vi "Control - Closed Loop Throttle.vi"(7 "Fresh Air Mass [mg/cyc]":sgl, 8 "Control Inputs":T1={"Engine Speed [RPM]"=0.0, "Engine Status"=enum."STALLED", "Load Control \nMode"=enum."High-Idle Governor", "dt(s)"=0.0, "Number of Cylinders"=0, "Engine Displacement [cc]"=0.0, "StoichAFR"=0.0, "Q.LHV Fuel [kJ/kg]"=0.0, "BattV PSU [V]"=0.0, "12V PSU [V]"=0.0, "5V PSU [V]"=0.0, "Pedal Position [%]"=0.0, "Oil Pressure [kPa]"=0.0, "Oil Temp [C]"=0.0, "Oil Level [%]"=0.0, "Engine Coolant Temp (ECT) [C]"=0.0, "Engine Coolant Pressure [kPa]"=0.0, "Rail Pressure [bar]"=0.0, "Fuel Pressure [kPa]"=0.0, "Fuel Temp [C]"=0.0, "Vacuum Pressure [kPa]"=0.0, "Throttle Position [%]"=0.0, "Cam1 Advance [CAD]"=0.0, "Cam2 Advance [CAD]"=0.0, "Cam3 Advance [CAD]"=0.0, "Cam4 Advance [CAD]"=0.0, "CA50 Control Output [CAD]"=[], "CA50 Control Output Valid"=[], "Intake Air Temp (IAT) [C]"=0.0, "Barometric Air Pressure [kPa]"=0.0, "Intake Air Rel. Humidity [%]"=0.0, "Mass Air Flow (MAF) [kg/hr]"=0.0, "Turbo Inlet Air Pressure [kPa]"=0.0, "Turbo Inlet Air Temp [C]"=0.0, "Turbo Outlet Air Pressure [kPa]"=0.0, "Turbo Outlet Air Temp [C]"=0.0, "CAC Outlet Pressure [kPa]"=0.0, "CAC Outlet Temp [C]"=0.0, "Intake Manifold Pressure (MAP) [kPa]"=0.0, "Intake Manifold Temp (MAT) [C]"=0.0, "Exhaust Manifold Pressure [kPa]"=0.0, "Exhaust Manifold Temp [C]"=0.0, "HighP EGR Cooler Outlet Pressure [kPa]"=0.0, "HighP EGR Cooler Outlet Temp [C]"=0.0, "HighP EGR Differential Pressure [kPa]"=0.0, "HighP EGR Valve Position [%]"=0.0, "Turbo Outlet Exhaust Pressure [kPa]"=0.0, "Turbo Outlet Exhaust Temp [C]"=0.0, "VGT Position 1 [%]"=0.0, "VGT Position 2 [%]"=0.0, "Turbo Speed 1 [RPM]"=0.0, "Turbo Speed 2 [RPM]"=0.0, "LowP EGR Differential Pressure [kPa]"=0.0, "LowP EGR Valve Position [%]"=0.0, "UEGO1Lambda"=0.0, "UEGO1_Hot"=FALSE, "UEGO2Lambda"=0.0, "UEGO2_Hot"=FALSE, "Knock Intensity"=[], "Knock"=[]} {"Knock Intensity" format="%.2f"; "CA50 Control Output [CAD]" format="%.2f"; "Exhaust Manifold Temp [C]" format="%#_6f"; "UEGO2Lambda" format="%.2f"; "Intake Manifold Temp (MAT) [C]" format="%#_6f"; "UEGO1Lambda" format="%.2f"}, 9 "Pedal [%]":sgl, 10 "Intake MAP Desired [kPa]":sgl, 11 "Fresh Air Mass Desired [mg/cyc]":sgl) -> (3 "Throttle Position [%Open]":sgl)   [LabVIEW 2015, in "ECS-RT.lvlib"]
uses:
  ECS-RT.lvlib
  Typedefs/Control Inputs/Control Inputs.ctl
  Typedefs/EPT/Engine Status.ctl
  Typedefs/MISC/Load Control Mode.ctl
  ECS-Shared.lvlib
panel:
  out "Pratio":sgl
  out "B1":sgl
  out "A1":sgl
  out "Pcr":sgl
  out "Psi":sgl
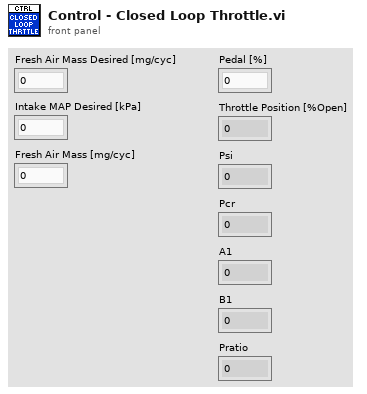
[diagram p1: front panel]
types:
  T1 = typedef "ECS-Shared.lvlib/Control Inputs.ctl" = cluster{"Engine Speed [RPM]":sgl, "Engine Status":T2, "Load Control \nMode":T3, "dt(s)":sgl, "Number of Cylinders":u8, "Engine Displacement [cc]":sgl, "StoichAFR":sgl, "Q.LHV Fuel [kJ/kg]":sgl, "BattV PSU [V]":sgl, "12V PSU [V]":sgl, "5V PSU [V]":sgl, "Pedal Position [%]":sgl, "Oil Pressure [kPa]":sgl, "Oil Temp [C]":sgl, "Oil Level [%]":sgl, "Engine Coolant Temp (ECT) [C]":sgl, "Engine Coolant Pressure [kPa]":sgl, "Rail Pressure [bar]":sgl, "Fuel Pressure [kPa]":sgl, "Fuel Temp [C]":sgl, "Vacuum Pressure [kPa]":sgl, "Throttle Position [%]":sgl, "Cam1 Advance [CAD]":sgl, "Cam2 Advance [CAD]":sgl, "Cam3 Advance [CAD]":sgl, "Cam4 Advance [CAD]":sgl, "CA50 Control Output [CAD]":sgl[], "CA50 Control Output Valid":bool[], "Intake Air Temp (IAT) [C]":sgl, "Barometric Air Pressure [kPa]":sgl, "Intake Air Rel. Humidity [%]":sgl, "Mass Air Flow (MAF) [kg/hr]":sgl, "Turbo Inlet Air Pressure [kPa]":sgl, "Turbo Inlet Air Temp [C]":sgl, "Turbo Outlet Air Pressure [kPa]":sgl, "Turbo Outlet Air Temp [C]":sgl, "CAC Outlet Pressure [kPa]":sgl, "CAC Outlet Temp [C]":sgl, "Intake Manifold Pressure (MAP) [kPa]":sgl, "Intake Manifold Temp (MAT) [C]":sgl, "Exhaust Manifold Pressure [kPa]":sgl, "Exhaust Manifold Temp [C]":sgl, "HighP EGR Cooler Outlet Pressure [kPa]":sgl, "HighP EGR Cooler Outlet Temp [C]":sgl, "HighP EGR Differential Pressure [kPa]":sgl, "HighP EGR Valve Position [%]":sgl, "Turbo Outlet Exhaust Pressure [kPa]":sgl, "Turbo Outlet Exhaust Temp [C]":sgl, "VGT Position 1 [%]":sgl, "VGT Position 2 [%]":sgl, "Turbo Speed 1 [RPM]":sgl, "Turbo Speed 2 [RPM]":sgl, "LowP EGR Differential Pressure [kPa]":sgl, "LowP EGR Valve Position [%]":sgl, "UEGO1Lambda":sgl, "UEGO1_Hot":bool, "UEGO2Lambda":sgl, "UEGO2_Hot":bool, "Knock Intensity":sgl[], "Knock":bool[]}
  T2 = typedef "ECS-Shared.lvlib/Engine Status.ctl" = enum16{"OFF", "STALLED", "CRANKING", "RUNNING", "ACCEL", "DECEL", "SAFE"}
  T3 = typedef "ECS-Shared.lvlib/Load Control Mode.ctl" = enum16{"No Governor", "Low-Idle Governor", "High-Idle Governor"}
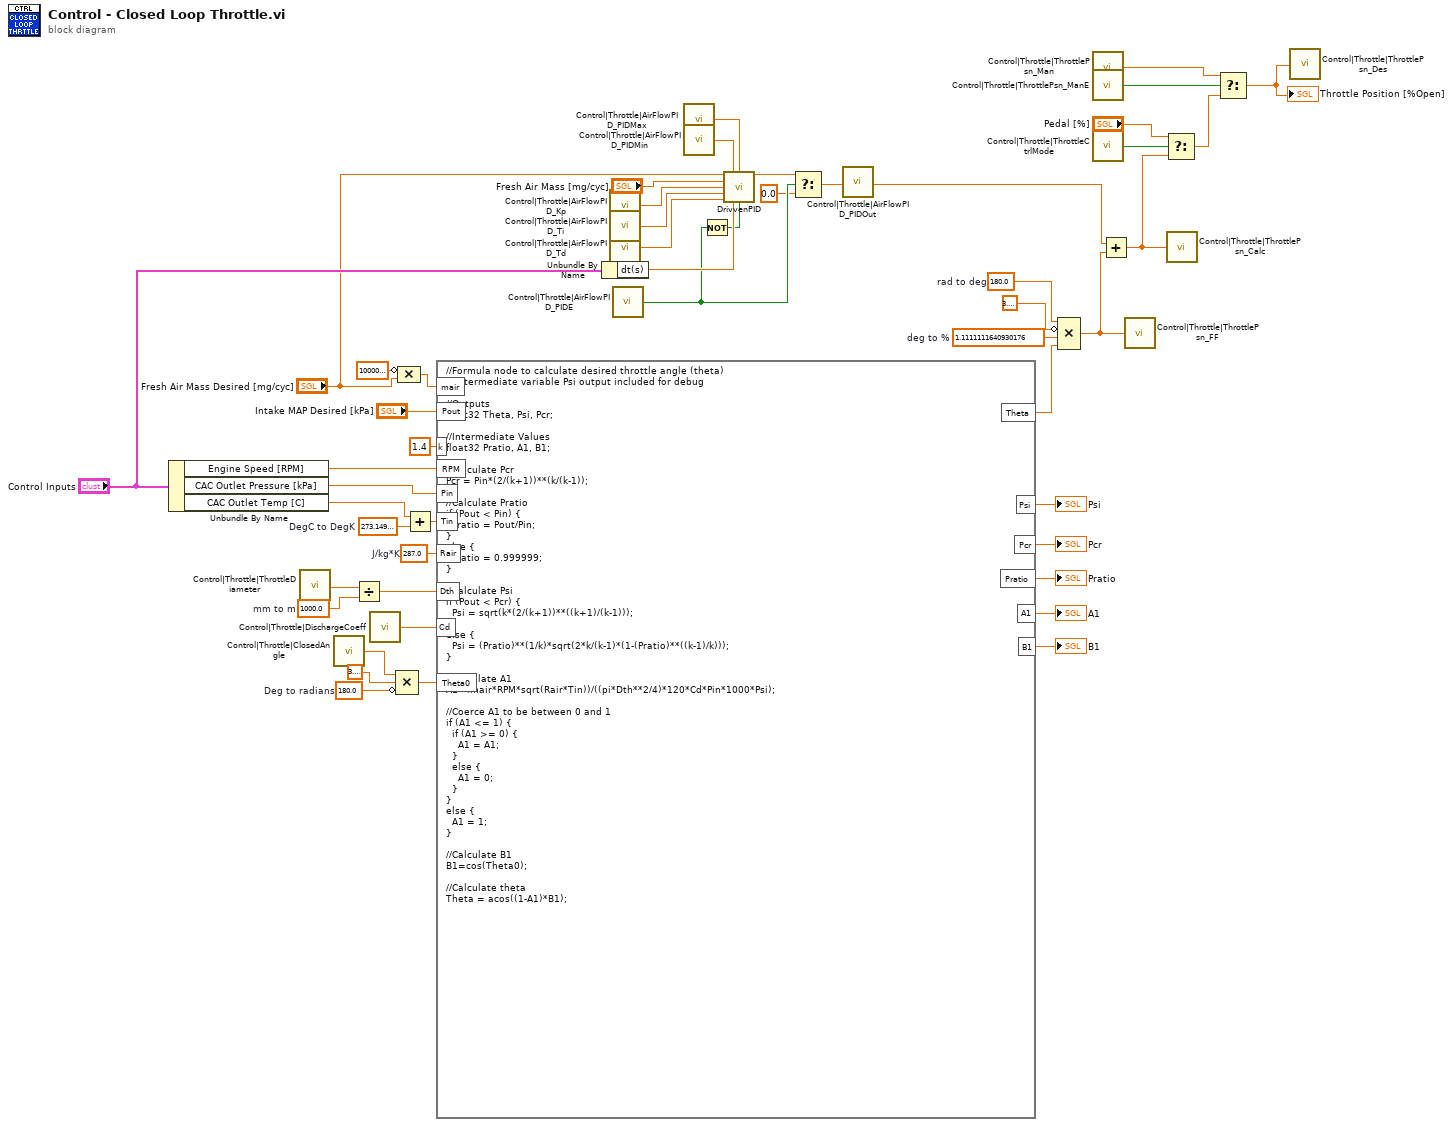
[diagram p0: block diagram]
diagram:
  w5 = sgl 180.0  # rad to deg
  w28 = sgl 1.1111112  # deg to %
  w32 = sgl 180.0  # Deg to radians
  w38 = sgl 1000.0  # mm to m
  w41 = sgl 273.15  # DegC to DegK
  w42 = 287.0  # J/kg*K
  n1 = Unbundle By Name("Control Inputs") -> ("Engine Speed [RPM]"=w33:sgl, "CAC Outlet Pressure [kPa]"=w10:sgl, "CAC Outlet Temp [C]"=w11:sgl)
  n2 = call "Control|Throttle|ThrottleDiameter"() -> ("Value"=w39:sgl)
  n3 = call "Control|Throttle|ClosedAngle"() -> ("Value"=w35:sgl)
  n4 = Divide(x=w39, y=w38) -> (x/y=w37:sgl)
  n5 = call "Control|Throttle|DischargeCoeff"() -> ("Value"=w36:sgl)
  n6 = Compound Arithmetic op=MULTIPLY(w35, sgl 3.1415927, invert w32) -> (w34:sgl)
  n7 = Compound Arithmetic op=MULTIPLY(invert sgl 1000000.0 ("value"), "Fresh Air Mass Desired [mg/cyc]") -> (w3:sgl)
  n8 = Add(x=w11, y=w41) -> (x+y=w40:sgl)
  n9 = formula code="//Formula node to calculate desired throttle angle (theta)\n// Intermediate variable Psi output included for debug\n\n//Outputs\nfloat32 Theta, Psi, Pcr;\n\n//Intermediate Values\nfloat32 Pratio, A1, B1;\n\n//Calculate Pcr\nPcr = Pin*(2/(k+1))**(k/(k-1));\n\n//Calculate Pratio\nif (Pout < Pin) {\n  Pratio = Pout/Pin;\n}\nelse {\n  Pratio = 0.999999;\n}\n\n//Calculate Psi\nif (Pout < Pcr) {\n  Psi = sqrt(k*(2/(k+1))**((k+1)/(k-1)));\n}\nelse {\n  Psi = (Pratio)**(1/k)*sqrt(2*k/(k-1)*(1-(Pratio)**((k-1)/k)));\n}\n\n//Calculate A1\nA1=(mair*RPM*sqrt(Rair*Tin))/((pi*Dth**2/4)*120*Cd*Pin*1000*Psi);\n\n//Coerce A1 to be between 0 and 1\nif (A1 <= 1) {\n  if (A1 >= 0) {\n    A1 = A1;\n  }\n  else {\n    A1 = 0;\n  }\n}\nelse {\n  A1 = 1;\n}\n\n//Calculate B1\nB1=cos(Theta0);\n\n//Calculate theta\nTheta = acos((1-A1)*B1);"("mair"=w3, "k"=1.4 ("input variable"), "Pin"=w10, "Pout"="Intake MAP Desired [kPa]", "Tin"=w40, "Rair"=w42, "Dth"=w37, "Cd"=w36, "Theta0"=w34, "RPM"=w33) -> ("Theta"=w27:sgl, "Psi"=→"Psi":sgl, "Pcr"=→"Pcr":sgl, "A1"=→"A1":sgl, "B1"=→"B1":sgl, "Pratio"=→"Pratio":sgl)
  n10 = Unbundle By Name("Control Inputs") -> ("dt(s)"=w22:sgl)
  n11 = call "Control|Throttle|AirFlowPID_Kp"() -> ("Value"=w25:sgl)
  n12 = call "Control|Throttle|AirFlowPID_Ti"() -> ("Value"=w24:sgl)
  n13 = call "Control|Throttle|AirFlowPID_Td"() -> ("Value"=w23:sgl)
  n14 = call "Control|Throttle|AirFlowPID_PIDE"() -> ("Value"=w20:bool)
  n15 = call "Control|Throttle|AirFlowPID_PIDMax"() -> ("Value"=w17:sgl)
  n16 = call "Control|Throttle|AirFlowPID_PIDMin"() -> ("Value"=w16:sgl)
  n17 = Not(x=w20) -> (.not. x?=w21:bool)
  n18 = call <vilib>:"DrivvenPID.vi"("Setpoint"="Fresh Air Mass Desired [mg/cyc]", "OutputLow"=w16, "OutputHigh"=w17, "ProcessVariable"="Fresh Air Mass [mg/cyc]", "ProportionalGain (Kc)"=w25, "IntegralTime (Ti, min)"=w24, "DerivativeTime (Td, min)"=w23, "dt (s)"=w22, "Reinitialize? (F)"=w21) -> ("Output"=w19:sgl)  [unwired: 1 in, 5 out]
  n19 = Select(t=w19, s=w20, f=sgl 0.0) -> (s? t:f=w13:sgl)
  n20 = call "Control|Throttle|AirFlowPID_PIDOut"("Value"=w13) -> ()
  n21 = Compound Arithmetic op=MULTIPLY(w5, invert sgl 3.1415927, w28, w27) -> (w14:sgl)
  n22 = call "Control|Throttle|ThrottlePsn_Man"() -> ("Value"=w48:sgl)
  n23 = call "Control|Throttle|ThrottlePsn_ManE"() -> ("Value"=w49:bool)
  n24 = call "Control|Throttle|ThrottleCtrlMode"() -> ("Value"=w47:bool)
  n25 = Add(x=w13, y=w14) -> (x+y=w15:sgl)
  n26 = call "Control|Throttle|ThrottlePsn_FF"("Value"=w14) -> ()
  n27 = Select(t="Pedal [%]", s=w47, f=w15) -> (s? t:f=w44:sgl)
  n28 = call "Control|Throttle|ThrottlePsn_Calc"("Value"=w15) -> ()
  n29 = Select(t=w48, s=w49, f=w44) -> (s? t:f=w45:sgl)
  "Throttle Position [%Open]" <- w45
  n30 = call "Control|Throttle|ThrottlePsn_Des"("Value"=w45) -> ()
